vi "test_struct_ads_surface_vapor.vi"() -> ()   [LabVIEW 2017]
doc: "Minimal example that demonstrates functions implemented in the SorpPropLib for adsorption working pairs based on the surface approach and using the vapor pressure as additional property."
panel:
  out "Der. of loading wrt. pressure":cluster{dbl[], dbl[]}[](graph)=[{[1000.0, 1001.0, 1002.0, 1003.0, 1004.0, 1005.0, 1006.0, 1007.0, 1008.0, 1009.0], [-1.0, -1.0, -1.0, -1.0, -1.0, -1.0, -1.0, -1.0, -1.0, -1.0]}, {[1000.0, 1001.0, 1002.0, 1003.0, 1004.0, 1005.0, 1006.0, 1007.0, 1008.0, 1009.0], [-1.0, -1.0, -1.0, -1.0, -1.0, -1.0, -1.0, -1.0, -1.0, -1.0]}]
  out "Der. of loading wrt. temperature":cluster{dbl[], dbl[]}[](graph)=[{[1000.0, 1001.0, 1002.0, 1003.0, 1004.0, 1005.0, 1006.0, 1007.0, 1008.0, 1009.0], [-1.0, -1.0, -1.0, -1.0, -1.0, -1.0, -1.0, -1.0, -1.0, -1.0]}, {[1000.0, 1001.0, 1002.0, 1003.0, 1004.0, 1005.0, 1006.0, 1007.0, 1008.0, 1009.0], [-1.0, -1.0, -1.0, -1.0, -1.0, -1.0, -1.0, -1.0, -1.0, -1.0]}]
  out "Der. of pressure wrt. loading":cluster{dbl[], dbl[]}[](graph)=[{[1000.0, 1001.0, 1002.0, 1003.0, 1004.0, 1005.0, 1006.0, 1007.0, 1008.0, 1009.0], [-1.0, -1.0, -1.0, -1.0, -1.0, -1.0, -1.0, -1.0, -1.0, -1.0]}, {[1000.0, 1001.0, 1002.0, 1003.0, 1004.0, 1005.0, 1006.0, 1007.0, 1008.0, 1009.0], [-1.0, -1.0, -1.0, -1.0, -1.0, -1.0, -1.0, -1.0, -1.0, -1.0]}]
  out "Der. of pressure wrt. temperature":cluster{dbl[], dbl[]}[](graph)=[{[1000.0, 1001.0, 1002.0, 1003.0, 1004.0, 1005.0, 1006.0, 1007.0, 1008.0, 1009.0], [-1.0, -1.0, -1.0, -1.0, -1.0, -1.0, -1.0, -1.0, -1.0, -1.0]}, {[1000.0, 1001.0, 1002.0, 1003.0, 1004.0, 1005.0, 1006.0, 1007.0, 1008.0, 1009.0], [-1.0, -1.0, -1.0, -1.0, -1.0, -1.0, -1.0, -1.0, -1.0, -1.0]}]
  out "Temperature":cluster{dbl[], dbl[]}[](graph)=[{[1000.0, 1001.0, 1002.0, 1003.0, 1004.0, 1005.0, 1006.0, 1007.0, 1008.0, 1009.0], [-1.0, -1.0, -1.0, -1.0, -1.0, -1.0, -1.0, -1.0, -1.0, -1.0]}, {[1000.0, 1001.0, 1002.0, 1003.0, 1004.0, 1005.0, 1006.0, 1007.0, 1008.0, 1009.0], [-1.0, -1.0, -1.0, -1.0, -1.0, -1.0, -1.0, -1.0, -1.0, -1.0]}]
  out "Pressure":cluster{dbl[], dbl[]}[](graph)=[{[1000.0, 1001.0, 1002.0, 1003.0, 1004.0, 1005.0, 1006.0, 1007.0, 1008.0, 1009.0], [-1.0, -1.0, -1.0, -1.0, -1.0, -1.0, -1.0, -1.0, -1.0, -1.0]}, {[1000.0, 1001.0, 1002.0, 1003.0, 1004.0, 1005.0, 1006.0, 1007.0, 1008.0, 1009.0], [-1.0, -1.0, -1.0, -1.0, -1.0, -1.0, -1.0, -1.0, -1.0, -1.0]}]
  out "Loading":cluster{dbl[], dbl[]}[](graph)=[{[1000.0, 1001.0, 1002.0, 1003.0, 1004.0, 1005.0, 1006.0, 1007.0, 1008.0, 1009.0], [-1.0, -1.0, -1.0, -1.0, -1.0, -1.0, -1.0, -1.0, -1.0, -1.0]}, {[1000.0, 1001.0, 1002.0, 1003.0, 1004.0, 1005.0, 1006.0, 1007.0, 1008.0, 1009.0], [-1.0, -1.0, -1.0, -1.0, -1.0, -1.0, -1.0, -1.0, -1.0, -1.0]}]
  in  "WorkingPair (Input)":T1={"no_iso"=1, "no_p_sat"=1, "path_db"="D:\\Driesel\\SorpLibLocal\\labview_wrapper\\data\\json\\sorpproplib.json", "wp_as"="silica gel pellet", "wp_st"="Fuji A", "wp_iso"="Freundlich", "wp_rf"="Water", "rf_rhol"="SaturatedLiquidDensity_EoS1", "no_rhol"=1, "rf_psat"="VaporPressure_EoS1"}
  in  "Temperature in K (Input)":dbl=300.0
  in  "Pressure in Pa (Input)":dbl=1000.0
  # "Increase pressure by 5000 Pa in steps of 1 Pa."
  # "Path to database"
  # "Name of sorbent"
  # "Name of sub-type of sorbent"
  # "Name of refrigerant"
  # "Name of isotherm"
  # "ID of isotherm"
  # "Name of calculation approach for vapor pressure"
  # "ID of vapor pressure equation"
  # "Name of calculation approach for liquid density"
  # "ID of liquid density equation"
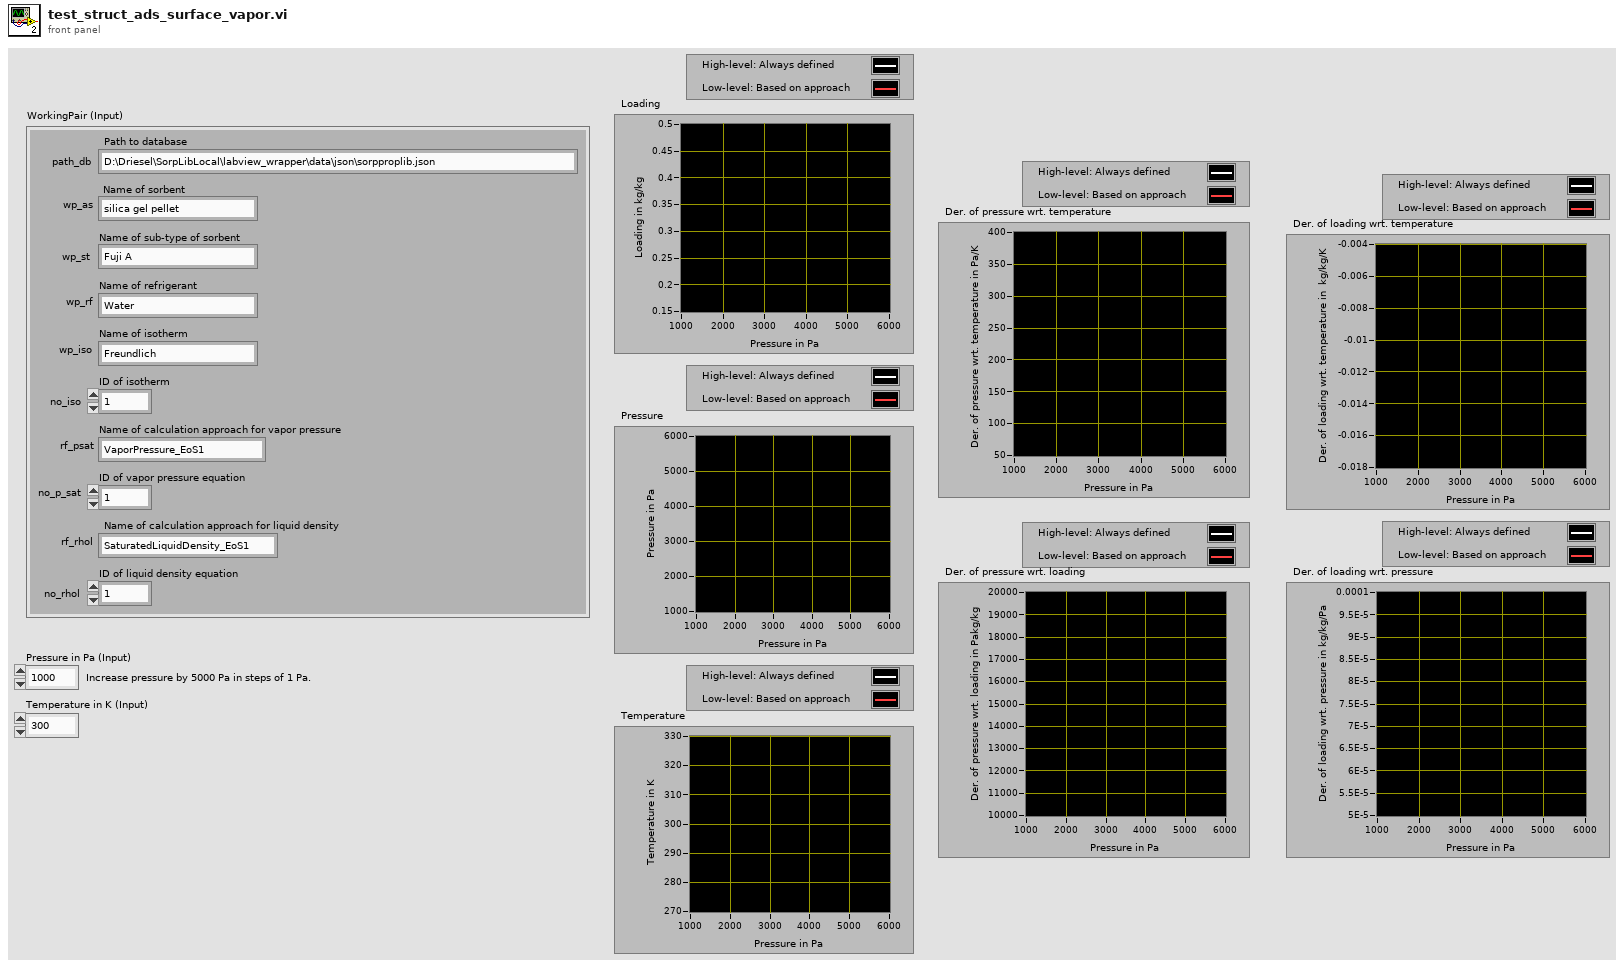
[diagram p1: front panel]
types:
  T1 = cluster{"no_iso":i32, "no_p_sat":i32, "path_db":string, "wp_as":string, "wp_st":string, "wp_iso":string, "wp_rf":string, "rf_rhol":string, "no_rhol":i32, "rf_psat":string}
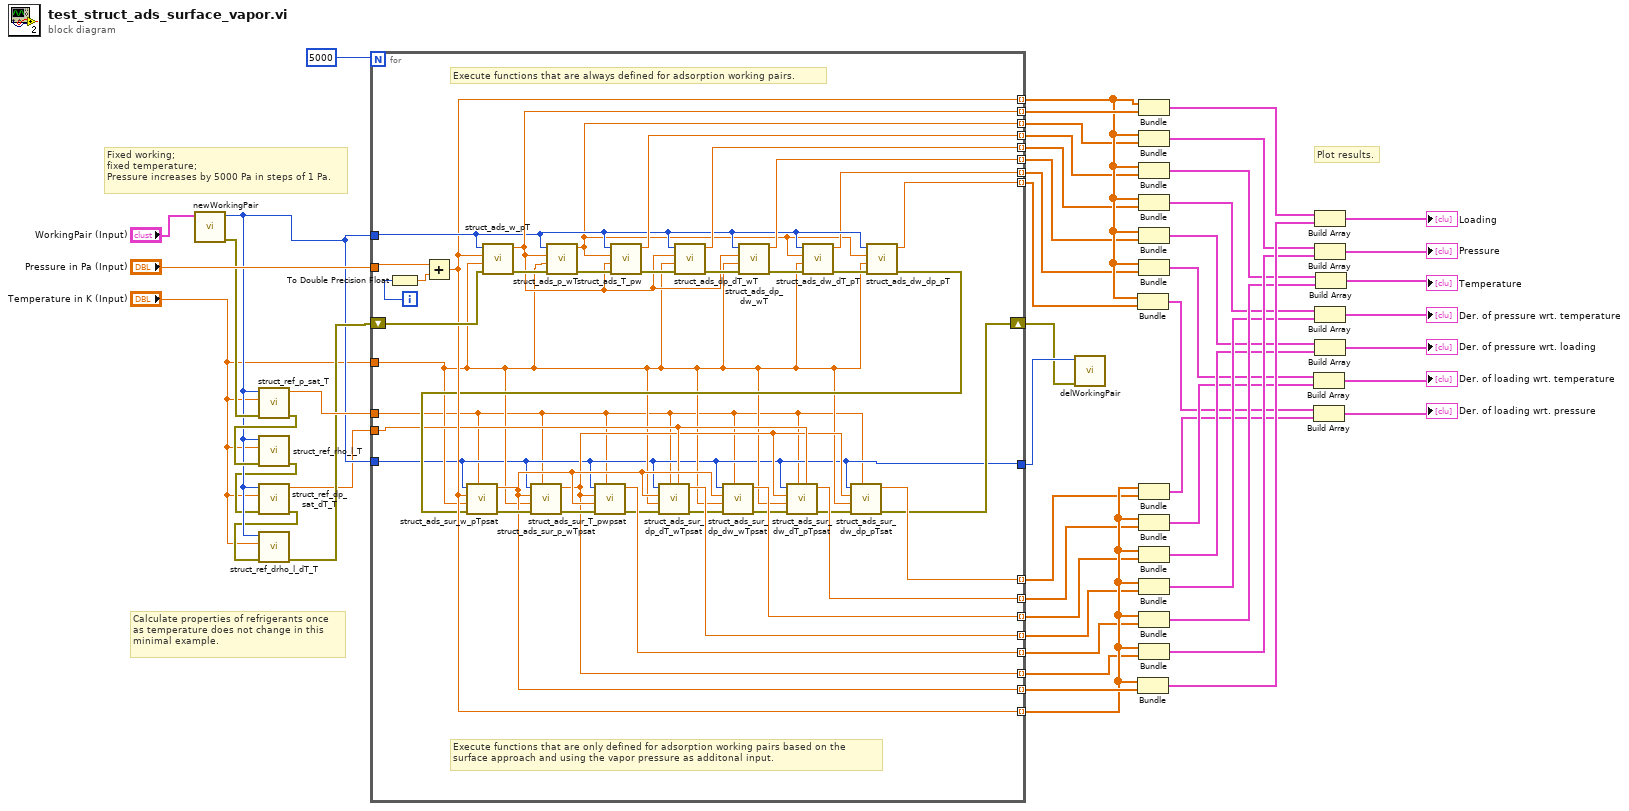
[diagram p0: block diagram]
diagram:
  # "Calculate properties of refrigerants once\nas temperature does not change in this\nminimal example."
  # "Plot results."
  # "Fixed working;\nfixed temperature;\nPressure increases by 5000 Pa in steps of 1 Pa."
  n1 = call "newWorkingPair.vi"("WorkingPair (Input)"="WorkingPair (Input)") -> ("Error (Output)"=w8:errorcluster, "workingPair"=w5:i64)  [unwired: 9 in]
  n2 = call "struct_ref_p_sat_T.vi"("Error (Input)"=w8, "Temperature in K (Input)"="Temperature in K (Input)", "Reference working pair (Input)"=w5) -> ("Error (Output)"=w7:errorcluster, "Saturation pressure in Pa (Output)"=w9:dbl)  [unwired: 7 in]
  n3 = call "struct_ref_rho_l_T.vi"("Error (Input)"=w7, "Temperature in K (Input)"="Temperature in K (Input)", "Reference working pair (Input)"=w5) -> ("Error (Output)"=w4:errorcluster)  [unwired: 7 in, 1 out]
  n4 = call "struct_ref_dp_sat_dT_T.vi"("Error (Input)"=w4, "Temperature in K (Input)"="Temperature in K (Input)", "Reference working pair (Input)"=w5) -> ("Error (Output)"=w3:errorcluster, "Der. of saturation pressure wrt temperature in Pa/K (Output)"=w1:dbl)  [unwired: 7 in]
  n5 = call "struct_ref_drho_l_dT_T.vi"("Error (Input)"=w3, "Temperature in K (Input)"="Temperature in K (Input)", "Reference working pair (Input)"=w5) -> ("Error (Output)"=w6:errorcluster)  [unwired: 7 in, 1 out]
  n6 = for {
    N: 5000 -> [_]
    tunnel: "Pressure in Pa (Input)" -> [w89]
    tunnel: "Temperature in K (Input)" -> [w56]
    tunnel: w5 -> [w75]
    shift-right: [w54] -> w10
    shift-left: w6 -> [w86]
    tunnel: [w84] -> w46 mode=indexing
    tunnel: [w71] -> w48 mode=indexing
    tunnel: [w77] -> w49 mode=indexing
    tunnel: [w72] -> w47 mode=indexing
    tunnel: [w82] -> w45 mode=indexing
    tunnel: [w79] -> w44 mode=indexing
    tunnel: [w74] -> w42 mode=indexing
    tunnel: [w73] -> w43 mode=indexing
    tunnel: w5 -> [w53]
    tunnel: [w63] -> w41 mode=indexing
    tunnel: [w71] -> w40 mode=indexing
    tunnel: [w57] -> w39 mode=indexing
    tunnel: [w67] -> w38 mode=indexing
    tunnel: [w65] -> w27 mode=indexing
    tunnel: [w62] -> w24 mode=indexing
    tunnel: [w59] -> w20 mode=indexing
    tunnel: [w58] -> w19 mode=indexing
    tunnel: [w53] -> w11
    tunnel: w9 -> [w52]
    tunnel: w1 -> [w60]
    i -> [w88]
    # "Execute functions that are only defined for adsorption working pairs based on the\nsurface approach and using the vapor pressure as additonal input."
    # "Execute functions that are always defined for adsorption working pairs."
    n7 = To Double Precision Float(number=w88) -> (double precision float=w87:dbl)
    n8 = Add(x=w89, y=w87) -> (x+y=w71:dbl)
    n9 = call "struct_ads_w_pT.vi"("Error (Input)"=w86, "Temperature in K (Input)"=w56, "Pressure in Pa (Input)"=w71, "Reference working pair (Input)"=w75) -> ("Error (Output)"=w85:errorcluster, "Loading in kg/kg (Output)"=w77:dbl)  [unwired: 6 in]
    n10 = call "struct_ads_p_wT.vi"("Error (Input)"=w85, "Temperature in K (Input)"=w56, "Loading in kg/kg (Input)"=w77, "Reference working pair (Input)"=w75) -> ("Error (Output)"=w83:errorcluster, "Pressure in Pa (Output)"=w72:dbl)  [unwired: 6 in]
    n11 = call "struct_ads_T_pw.vi"("Error (Input)"=w83, "Loading in kg/kg (Input)"=w77, "Pressure in Pa (Input)"=w72, "Reference working pair (Input)"=w75) -> ("Error (Output)"=w81:errorcluster, "Temperature in K (Output)"=w84:dbl)  [unwired: 6 in]
    n12 = call "struct_ads_dp_dT_wT.vi"("Error (Input)"=w81, "Temperature in K (Input)"=w56, "Loading in kg/kg (Input)"=w77, "Reference working pair (Input)"=w75) -> ("Error (Output)"=w80:errorcluster, "Der. of pressure wrt. temperature in Pa/K (Output)"=w82:dbl)  [unwired: 6 in]
    n13 = call "struct_ads_dp_dw_wT.vi"("Error (Input)"=w80, "Temperature in K (Input)"=w56, "Loading in kg/kg (Input)"=w77, "Reference working pair (Input)"=w75) -> ("Error (Output)"=w78:errorcluster, "Der. of pressure wrt. loading in Pakg/kg (Output)"=w79:dbl)  [unwired: 6 in]
    n14 = call "struct_ads_dw_dT_pT.vi"("Error (Input)"=w78, "Temperature in K (Input)"=w56, "Pressure in Pa (Input)"=w72, "Reference working pair (Input)"=w75) -> ("Error (Output)"=w76:errorcluster, "Der. of loading wrt. temperature in kg/kg/K (Output)"=w74:dbl)  [unwired: 6 in]
    n15 = call "struct_ads_dw_dp_pT.vi"("Error (Input)"=w76, "Temperature in K (Input)"=w56, "Pressure in Pa (Input)"=w72, "Reference working pair (Input)"=w75) -> ("Error (Output)"=w70:errorcluster, "Der. of loading wrt. pressure in kg/kg/Pa (Output)"=w73:dbl)  [unwired: 6 in]
    n16 = call "struct_ads_sur_w_pTpsat.vi"("Saturation vapor pressure in Pa (Input)"=w52, "Error (Input)"=w70, "Temperature in K (Input)"=w56, "Pressure in Pa (Input)"=w71, "Reference working pair (Input)"=w53) -> ("Error (Output)"=w69:errorcluster, "Equilibrium loading in kg/kg (Output)"=w63:dbl)  [unwired: 5 in]
    n17 = call "struct_ads_sur_p_wTpsat.vi"("Saturation vapor pressure in Pa (Input)"=w52, "Error (Input)"=w69, "Temperature in K (Input)"=w56, "Loading in kg/kg (Input)"=w63, "Reference working pair (Input)"=w53) -> ("Error (Output)"=w68:errorcluster, "Equilibrium pressure in Pa (Output)"=w57:dbl)  [unwired: 5 in]
    n18 = call "struct_ads_sur_T_pwpsat.vi"("Saturation vapor pressure in Pa (Input)"=w52, "Error (Input)"=w68, "Loading in kg/kg (Input)"=w63, "Pressure in Pa (Input)"=w57, "Reference working pair (Input)"=w53) -> ("Error (Output)"=w66:errorcluster, "Equilibrium temperature in K (Output)"=w67:dbl)  [unwired: 5 in]
    n19 = call "struct_ads_sur_dp_dT_wTpsat.vi"("Der. of saturation pressure wrt. temperature in Pa/K (Input)"=w60, "Saturation vapor pressure in Pa (Input)"=w52, "Error (Input)"=w66, "Temperature in K (Input)"=w56, "Loading in kg/kg (Input)"=w63, "Reference working pair (Input)"=w53) -> ("Error (Output)"=w64:errorcluster, "Der. pressure wrt. temperature in Pa/K (Output)"=w65:dbl)  [unwired: 4 in]
    n20 = call "struct_ads_sur_dp_dw_wTpsat.vi"("Saturation vapor pressure in Pa (Input)"=w52, "Error (Input)"=w64, "Temperature in K (Input)"=w56, "Loading in kg/kg (Input)"=w63, "Reference working pair (Input)"=w53) -> ("Error (Output)"=w61:errorcluster, "Der. pressure wrt. loading in Pakg/kg (Output)"=w62:dbl)  [unwired: 5 in]
    n21 = call "struct_ads_sur_dw_dT_pTpsat.vi"("Der. of saturation pressure wrt. temperature in Pa/K (Input)"=w60, "Saturation vapor pressure in Pa (Input)"=w52, "Error (Input)"=w61, "Temperature in K (Input)"=w56, "Pressure in Pa (Input)"=w57, "Reference working pair (Input)"=w53) -> ("Error (Output)"=w55:errorcluster, "Der. loading wrt. tempreature in kg/kg/K (Output)"=w59:dbl)  [unwired: 4 in]
    n22 = call "struct_ads_sur_dw_dp_pTsat.vi"("Saturation vapor pressure in Pa (Input)"=w52, "Error (Input)"=w55, "Temperature in K (Input)"=w56, "Pressure in Pa (Input)"=w57, "Reference working pair (Input)"=w53) -> ("Error (Output)"=w54:errorcluster, "Der. of loading wrt. pressure in kg/kg/Pa (Output)"=w58:dbl)  [unwired: 5 in]
  }
  n23 = call "delWorkingPair.vi"("Error (Input)"=w10, "workingPair"=w11) -> ()  [unwired: 9 in, 1 out]
  n24 = Bundle(w48, w43) -> (w16:cluster{dbl[], dbl[]})  [unwired: 1 in]
  n25 = Bundle(w40, w41) -> (w36:cluster{dbl[], dbl[]})  [unwired: 1 in]
  n26 = Bundle(w48, w49) -> (w37:cluster{dbl[], dbl[]})  [unwired: 1 in]
  n27 = Bundle(w48, w47) -> (w35:cluster{dbl[], dbl[]})  [unwired: 1 in]
  n28 = Bundle(w48, w46) -> (w33:cluster{dbl[], dbl[]})  [unwired: 1 in]
  n29 = Bundle(w48, w45) -> (w31:cluster{dbl[], dbl[]})  [unwired: 1 in]
  n30 = Bundle(w48, w44) -> (w23:cluster{dbl[], dbl[]})  [unwired: 1 in]
  n31 = Bundle(w48, w42) -> (w18:cluster{dbl[], dbl[]})  [unwired: 1 in]
  n32 = Bundle(w40, w19) -> (w15:cluster{dbl[], dbl[]})  [unwired: 1 in]
  n33 = Bundle(w40, w20) -> (w17:cluster{dbl[], dbl[]})  [unwired: 1 in]
  n34 = Bundle(w40, w24) -> (w22:cluster{dbl[], dbl[]})  [unwired: 1 in]
  n35 = Bundle(w40, w27) -> (w26:cluster{dbl[], dbl[]})  [unwired: 1 in]
  n36 = Bundle(w40, w38) -> (w32:cluster{dbl[], dbl[]})  [unwired: 1 in]
  n37 = Bundle(w40, w39) -> (w34:cluster{dbl[], dbl[]})  [unwired: 1 in]
  n38 = Build Array(w18, w17) -> (→"Der. of loading wrt. temperature":cluster{dbl[], dbl[]}[])
  n39 = Build Array(w16, w15) -> (→"Der. of loading wrt. pressure":cluster{dbl[], dbl[]}[])
  n40 = Build Array(w37, w36) -> (→"Loading":cluster{dbl[], dbl[]}[])
  n41 = Build Array(w35, w34) -> (→"Pressure":cluster{dbl[], dbl[]}[])
  n42 = Build Array(w31, w26) -> (→"Der. of pressure wrt. temperature":cluster{dbl[], dbl[]}[])
  n43 = Build Array(w23, w22) -> (→"Der. of pressure wrt. loading":cluster{dbl[], dbl[]}[])
  n44 = Build Array(w33, w32) -> (→"Temperature":cluster{dbl[], dbl[]}[])
